vi "Periodic Tasks.vi"(8 "error in":errorcluster) -> ()   [LabVIEW 2017]
doc: "This VI runs in parallel to other robot code. It can contain as many user-defined periodic loops as you need. These can carry out PID or other sorts of timed response."
uses:
  <vilib>/Rock Robotics/WPI/Utilities/WPI_GetSetVariantRefNum.vi
  Robot Global Data.vi
  <vilib>/Rock Robotics/Network Tables/NT Write Number.vi
  <vilib>/Rock Robotics/Network Tables/NT Write Boolean.vi
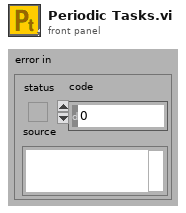
[diagram p1: front panel]
types:
  T1 = typedef "WPI_JoystickDevRef.ctl" = cluster{"Device":T2}
  T2 = typedef "WPI_JoystickDeviceEnum.ctl" = enum16{"USB 0", "USB 1", "USB 2", "USB 3", "USB 4", "USB 5"}
  T3 = typedef "WPI_GyroDevRef.ctl" = cluster{"DevStatus":errorcluster, "Analog Channel":T4, "Gain (VoltsPerDegree/Second)":dbl, "Gyro Type":enum16{"Analog", "XRS450"}, "Handle":i32, "SPI Bus":T5, "Device Found":bool, "Sample Rate":dbl, "Calibrate On Open":bool, "Offset":dbl}
  T4 = typedef "FPGA_AIChannel.ctl" = enum8{"AI 0", "AI 1", "AI 2", "AI 3", "AI MXP 0", "AI MXP 1", "AI MXP 2", "AI MXP 3", "Invalid"}
  T5 = typedef "spi_bus.ctl" = enum16{"SPI On-Board, CS0", "SPI On-Board, CS1", "SPI On-Board, CS2", "SPI On-Board, CS3", "SPI MXP", "Invalid"}
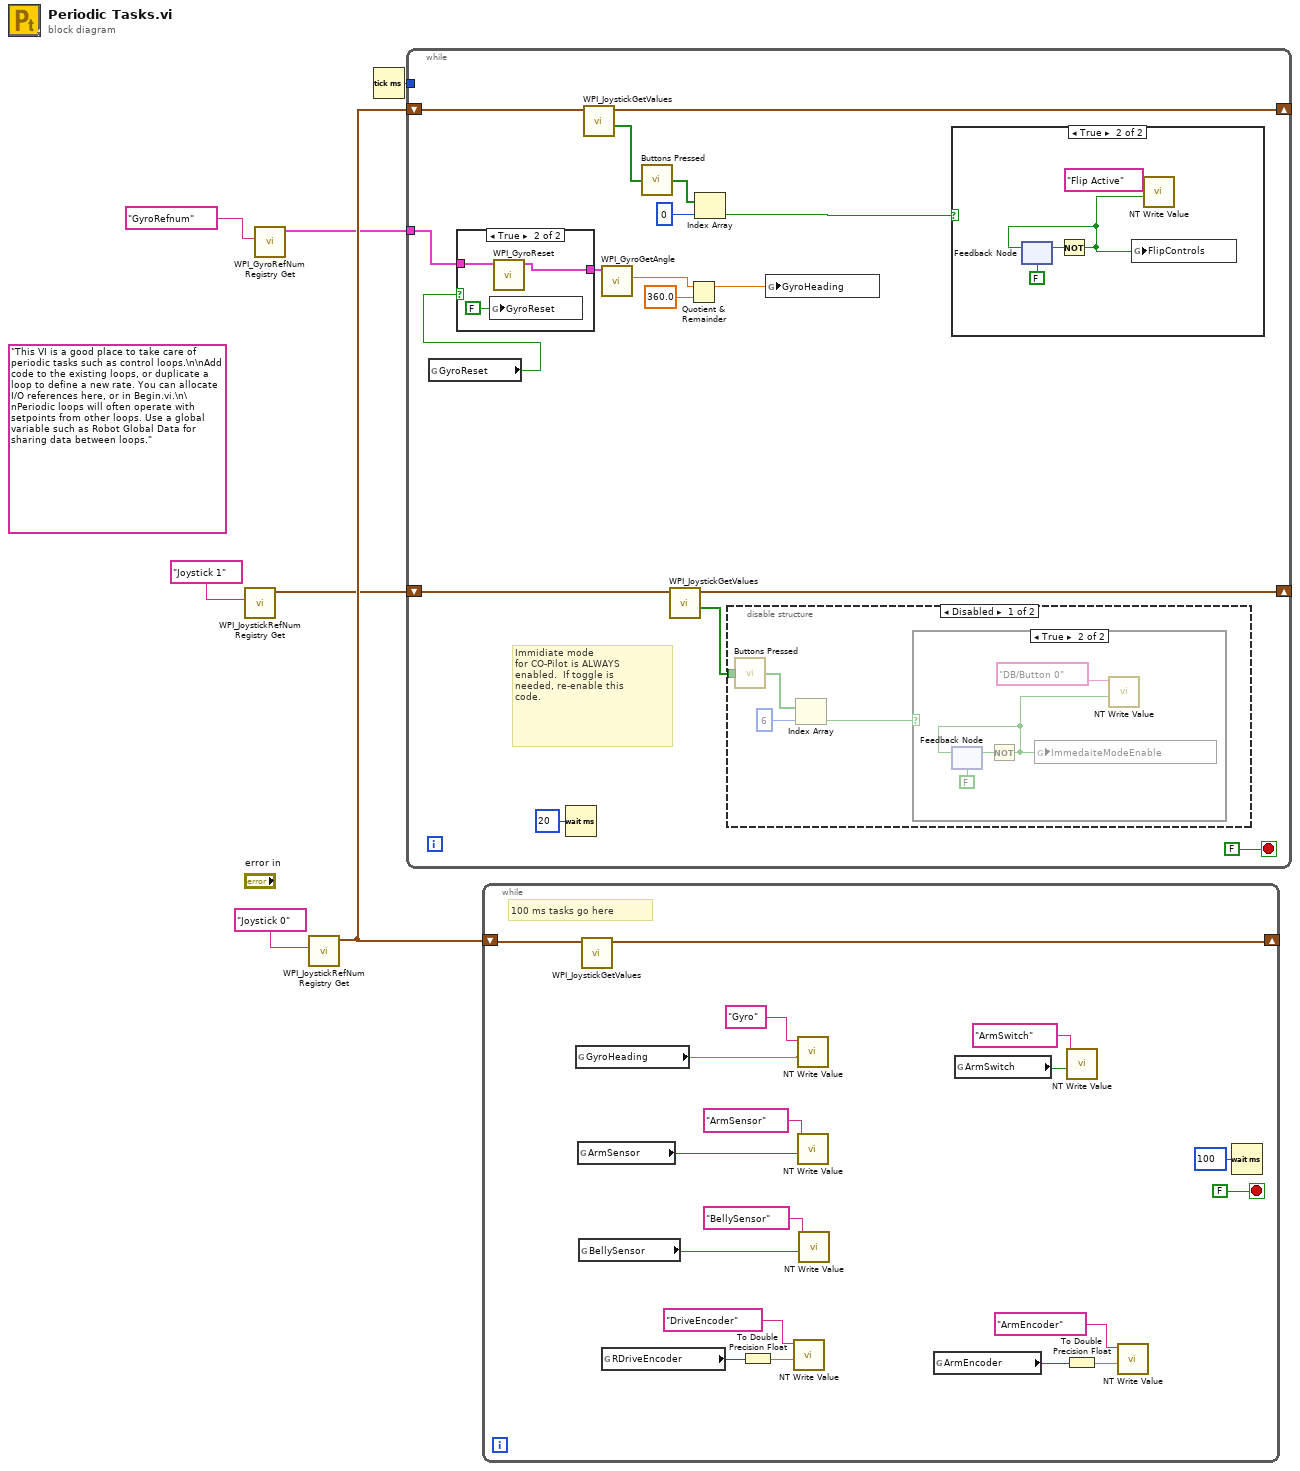
[diagram p0: block diagram]
diagram:
  (unwired) "This VI is a good place to take care of periodic tasks such as control loops.\n\nAdd code to the existing loops, or duplicate a loop to define a new rate. You can allocate I/O references here, or in Begin.vi.\n\nPeriodic loops will often operate with setpoints from other loops. Use a global variable such as Robot Global Data for sharing data between loops."
  n1 = call <vilib>:"WPI_JoystickRefNum Registry Get.vi"("refnum name"="Joystick 1") -> ("JoystickDevRef"=w1:T1)  [unwired: 1 in, 9 out]
  n2 = call <vilib>:"WPI_GyroRefNum Registry Get.vi"("refnum name"="GyroRefnum") -> ("GyroDevRef"=w3:T3)  [unwired: 9 in, 1 out]
  n3 = call <vilib>:"WPI_JoystickRefNum Registry Get.vi"("refnum name"="Joystick 0") -> ("JoystickDevRef"=w6:T1)  [unwired: 1 in, 9 out]
  n4 = Tick Count (ms)() -> (millisecond timer value=w5:u32)
  n5 = while {
    shift-right: [w18] -> _
    shift-left: w6 -> [w19]
    tunnel: w5 -> [_]
    tunnel: w3 -> [w11]
    shift-right: [w9] -> _
    shift-left: w1 -> [w10]
    stop <- FALSE stop-if-true
    # "Immidiate mode\nfor CO-Pilot is ALWAYS\nenabled.  If toggle is\nneeded, re-enable this\ncode."
    n6 = global read "Robot Global Data.vi" "GyroReset"() -> (w13:bool)
    n7 = case shown="True" w13 {
      tunnel: [w33 w35] -> w12
      tunnel: w11 -> [w33 w34]
      frame False {
      }
      frame True {
        n8 = global write "Robot Global Data.vi" "GyroReset"(FALSE ("GyroReset")) -> ()
        n9 = call <vilib>:"WPI_GyroReset.vi"("GyroDevRef"=w34) -> ("GyroDevRef"=w35:T3)  [unwired: 9 in, 1 out]
      }
    }
    n10 = Wait (ms)(milliseconds to wait=u32 20) -> ()  [unwired: 1 out]
    n11 = call <vilib>:"WPI_JoystickGetValues.vi"("JoystickDevRef"=w19) -> ("Buttons"=w21:bool[], "JoystickDevRef"=w18:T1)  [unwired: 6 in, 3 out]
    n12 = call <vilib>:"WPI_GyroGetAngle.vi"("GyroDevRef"=w12) -> ("Angle"=w15:dbl)  [unwired: 6 in, 4 out]
    n13 = call "Buttons Pressed.vi"("Button Values"=w21) -> ("Button Presses"=w20:bool[])
    n14 = call <vilib>:"WPI_JoystickGetValues.vi"("JoystickDevRef"=w10) -> ("Buttons"=w8:bool[], "JoystickDevRef"=w9:T1)  [unwired: 6 in, 3 out]
    n15 = Quotient & Remainder(x=w15, y=360.0) -> (x-y*floor(x/y)=w14:dbl)  [unwired: 1 out]
    n16 = Index Array(array=w20, index=0) -> (element=w17:bool)
    n17 = disable-structure shown="Disabled" {
      disable-tunnel: w8 -> [w26 _]
      frame Disabled {
        n18 = call "Buttons Pressed.vi"("Button Values"=w26) -> ("Button Presses"=w28:bool[])
        n19 = Index Array(array=w28, index=6) -> (element=w25:bool)
        n20 = case shown="True" w25 {
          frame False {
          }
          frame True {
            n21 = feedback #1(FALSE) -> (w30:bool)
            n22 = Not(x=w30) -> (.not. x?=w29:bool)
            n23 = feedback-in #1(w29) -> ()
            n24 = global write "Robot Global Data.vi" "ImmedaiteModeEnable"(w29) -> ()
            n25 = call-poly <vilib>:"NT Write Value.vi"("Boolean"=w29, "Name"="DB/Button 0") -> ()  [unwired: 9 in, 1 out]
          }
        }
      }
      frame Enabled {
      }
    }
    n26 = global write "Robot Global Data.vi" "GyroHeading"(w14) -> ()
    n27 = case shown="True" w17 {
      frame False {
      }
      frame True {
        n28 = feedback #2(FALSE) -> (w38:bool)
        n29 = Not(x=w38) -> (.not. x?=w37:bool)
        n30 = feedback-in #2(w37) -> ()
        n31 = global write "Robot Global Data.vi" "FlipControls"(w37) -> ()
        n32 = call-poly <vilib>:"NT Write Value.vi"("Boolean"=w37, "Name"="Flip Active") -> ()  [unwired: 9 in, 1 out]
      }
    }
  }
  n33 = while {
    shift-right: [w55] -> _
    shift-left: w6 -> [w56]
    stop <- FALSE stop-if-true
    # "100 ms tasks go here"
    n34 = global read "Robot Global Data.vi" "GyroHeading"() -> (w54:dbl)
    n35 = global read "Robot Global Data.vi" "ArmSensor"() -> (w52:bool)
    n36 = global read "Robot Global Data.vi" "BellySensor"() -> (w49:bool)
    n37 = call <vilib>:"WPI_JoystickGetValues.vi"("JoystickDevRef"=w56) -> ("JoystickDevRef"=w55:T1)  [unwired: 6 in, 4 out]
    n38 = global read "Robot Global Data.vi" "RDriveEncoder"() -> (w47:i32)
    n39 = To Double Precision Float(number=w47) -> (double precision float=w46:dbl)
    n40 = call-poly <vilib>:"NT Write Value.vi"("Numeric"=w46, "Name"="DriveEncoder") -> ()  [unwired: 9 in, 1 out]
    n41 = call-poly <vilib>:"NT Write Value.vi"("Numeric"=w54, "Name"="Gyro") -> ()  [unwired: 9 in, 1 out]
    n42 = call-poly <vilib>:"NT Write Value.vi"("Boolean"=w52, "Name"="ArmSensor") -> ()  [unwired: 9 in, 1 out]
    n43 = call-poly <vilib>:"NT Write Value.vi"("Boolean"=w49, "Name"="BellySensor") -> ()  [unwired: 9 in, 1 out]
    n44 = global read "Robot Global Data.vi" "ArmEncoder"() -> (w44:i32)
    n45 = global read "Robot Global Data.vi" "ArmSwitch"() -> (w42:bool)
    n46 = call-poly <vilib>:"NT Write Value.vi"("Boolean"=w42, "Name"="ArmSwitch") -> ()  [unwired: 9 in, 1 out]
    n47 = To Double Precision Float(number=w44) -> (double precision float=w43:dbl)
    n48 = call-poly <vilib>:"NT Write Value.vi"("Numeric"=w43, "Name"="ArmEncoder") -> ()  [unwired: 9 in, 1 out]
    n49 = Wait (ms)(milliseconds to wait=u32 100) -> ()  [unwired: 1 out]
  }
